vi "Verify Compass Data.vi"(1 "Compass Data":dbl) -> (0 "Data OK?":bool)   [LabVIEW 2009]
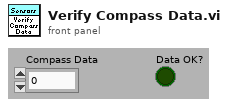
[diagram p1: front panel]
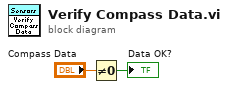
[diagram p0: block diagram]
diagram:
  n1 = Not Equal To 0?(x="Compass Data") -> (x != 0?=→"Data OK?":bool)
